vi "SendPosition.vi"(6 "error in":errorcluster, 9 "VISA resource In":refnum<visa-resource-name>) -> (0 "error out":errorcluster, 3 "VISA resource name out":refnum<visa-resource-name>)   [LabVIEW 2016]
panel:
  in  "Motor Position":dbl[](array[numeric])
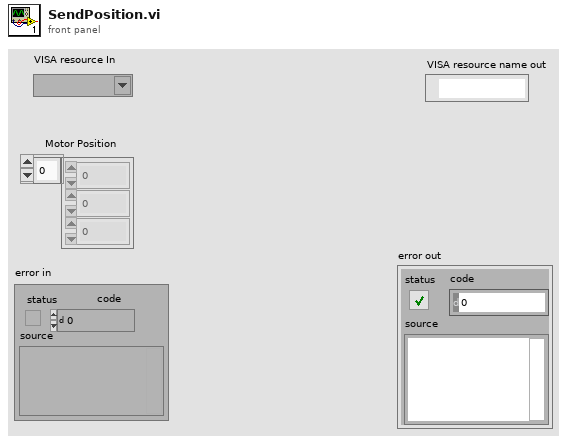
[diagram p1: front panel]
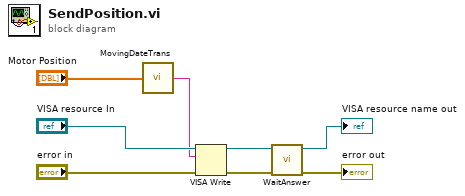
[diagram p0: block diagram]
diagram:
  n1 = call "MovingDateTrans.vi"("INPUT"="Motor Position") -> ("MOVEING COMMAND"=w6:string)  [unwired: 2 in]
  n2 = VISA Write(VISA resource name="VISA resource In", write buffer=w6, error in (no error)="error in") -> (VISA resource name out=w5:refnum<visa-resource-name>, error out=w3:errorcluster)  [unwired: 1 out]
  n3 = call "WaitAnswer.vi"("error in (no error)"=w3, "VISA resource name in"=w5) -> ("error out"=→"error out":errorcluster, "VISA resource name out"=→"VISA resource name out":refnum<visa-resource-name>)  [unwired: 4 in]
